vi "controllerTest.vi"() -> ()   [LabVIEW 2018]
panel:
  in  "Boolean":bool=TRUE
  in  "Tab Control 2":enum32{"Page 1", "Page 2"}(tab)
  in  "Tab Control":enum32{"Page 0", "Page 1"}(tab)
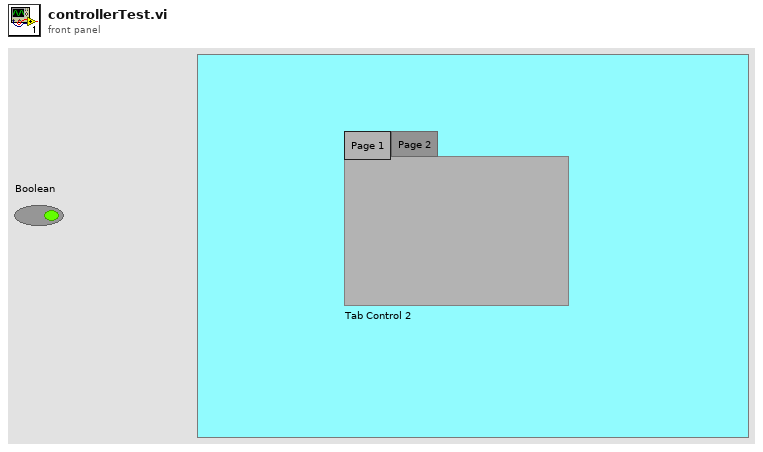
[diagram p1: front panel]
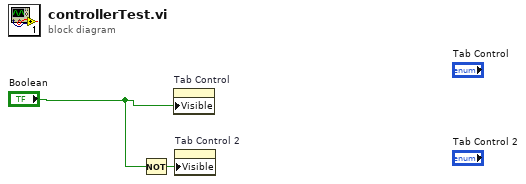
[diagram p0: block diagram]
diagram:
  n1 = Not(x="Boolean") -> (.not. x?=w2:bool)
  n2 = property on="Tab Control" class="TabCtl (strict)"("Visible"="Boolean") -> ()  [unwired: 2 in, 2 out]
  n3 = property on="Tab Control 2" class="TabCtl (strict)"("Visible"=w2) -> ()  [unwired: 2 in, 2 out]
